vi "lxw name to row 2.vi"(8 "error in (no error)":errorcluster, 11 "row_str":string) -> (0 "error out":errorcluster, 3 "function return":u32)   [LabVIEW 2015, in "xlsxwriter.lvlib"]
doc: "uint32_t lxw_name_to_row_2(const char *row_str);"
uses:
  xlsxwriter.lvlib
  xlsxwriter.dll
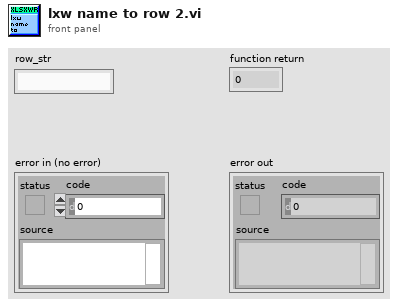
[diagram p1: front panel]
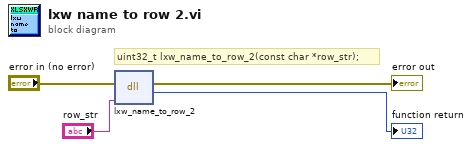
[diagram p0: block diagram]
diagram:
  # "uint32_t lxw_name_to_row_2(const char *row_str);"
  n1 = dll-call lib="C:/Users/WDAGUtilityAccount/Desktop/lv_vis_added_cell/xlsxwriter.*" fn="lxw_name_to_row_2"(error in="error in (no error)", "row_str"="row_str") -> (error out=→"error out":errorcluster, →"function return":u32)  [unwired: 3 in, 1 out]
